vi "MovementModel.vi"(0 "Start Vector":T3, 2 "Destination":cluster{"x":dbl, "y":dbl}, 3 "Log All Points":bool, 5 "Segment Length (m)":dbl=0.1, 8 "Do Force Direction":bool, 9 "Movement Settings":T2={"Arrival Tolerance (m)"=0.01, "Closeness Threshold (m)"=0.5, "Pit Obstacle Radius (m)"=0.5, "Pit Locations"=[]}, 10 "Turn Radius (m)":dbl=1.7, 11 "Force Direction Forward (If Forcing)":bool) -> (15 "Move":T1, 18 "Final Position":cluster{"x":dbl, "y":dbl, "angle":dbl})   [LabVIEW 2015, in "Navigation2017.lvlib"]
doc: "Closeness Threshold is used to calculate closeness of each robot corner to walls and obstacles, which is summed and returned as Closeness Sum (a value used in path scoring).\n\nFrom lua prototype:\n--[[\nIteratively moves the robot along a circular/straight curve towards the \nend point. This movement may or may not succeed, and the result is given\nin didReach. The \"resolution\" of the movement is determined by segLength,\nin meters/iteration of movement. The movement will also fail if the robot \ncollides with the edge of the arena. \n\nThe robot may move forward or backward, depending on the closer of the \nsummed distances of the cameras on the front and back.\n\nTurning radius is determined by the variable provided above.\n\nlogAllPoints defaults to false\n \nParams:\n startX, startY - in meters\n startAngle - in rads\n destX, destY - destination point\n (you cannot specify an end angle, fundamentally)\n logAllPoints - for animation and rendering. defaults to false if set to nil\n forceDirection - force robot to move forwards or backwards. nil lets closer end \n of robot determine. Forwards = true, backwards = false if you do set this\n value.\n\nReturns a movement table:\n- didReach\n- didCollide\n- angleSum (how many radians robot turned over course of movement)\n- length (sum length of segments)\n- closeness (closeness of robot to walls and pits. should be mostly independent of segLength)\n- array of positions: (either just a couple or many, depending on logAllPoints)\n - {x, y, angle}\n- movedFwd (boolean)\n--]]"
uses:
  Navigation2017.lvlib
  Vector.ctl
  MovementSettings.ctl
  Move.ctl
  <vilib>/Analysis/coordinate.llb/Angle Range (Degree).ctl
  <vilib>/Analysis/coordinate.llb/Wrap Angle (scalar).vi
  Navigation2017-SubVIs.lvlib
  Navigation2017-util.lvlib
  <vilib>/Analysis/NI_AAL_Angle.lvlib
panel:
  # "OUTPUTS"
  # "INPUTS"
  # "Analogous to \nmovementmodel.lua -> move()"
  # "--[[\nIteratively moves the robot along a circular/straight curve towards the \nend point. This movement may or may not succeed, and the result is given\nin didReach. The \"resolution\" of the movement is determined by segLength,\nin meters/iteration of movement. The movement will also fail if the robot \ncollides with the edge of the arena. \n\nThe robot may move forward or backward, depending on the closer of the \nsummed distances of the cameras on the front and back.\n\nTurning radius is determined by the variable provided above.\n\nlogAllPoints defaults to false\n    \nParams:\n  startX, startY - in meters\n  startAngle - in rads\n  destX, destY - destination point\n    (you cannot specify an end angle, fundamentally)\n  logAllPoints - for animation and rendering. defaults to false if set to nil\n  forceDirection - force robot to move forwards or backwards. nil lets closer end \n    of robot determine. Forwards = true, backwards = false if you do set this\n    value.\n\nReturns a movement table:\n- didReach\n- didCollide\n- angleSum (how many radians robot turned over course of movement)\n- length (sum length of segments)\n- closeness (closeness of robot to walls and pits. should be mostly independent of segLength)\n- array of positions: (either just a couple or many, depending on logAllPoints)\n  - {x, y, angle}\n- movedFwd (boolean)\n--]]"
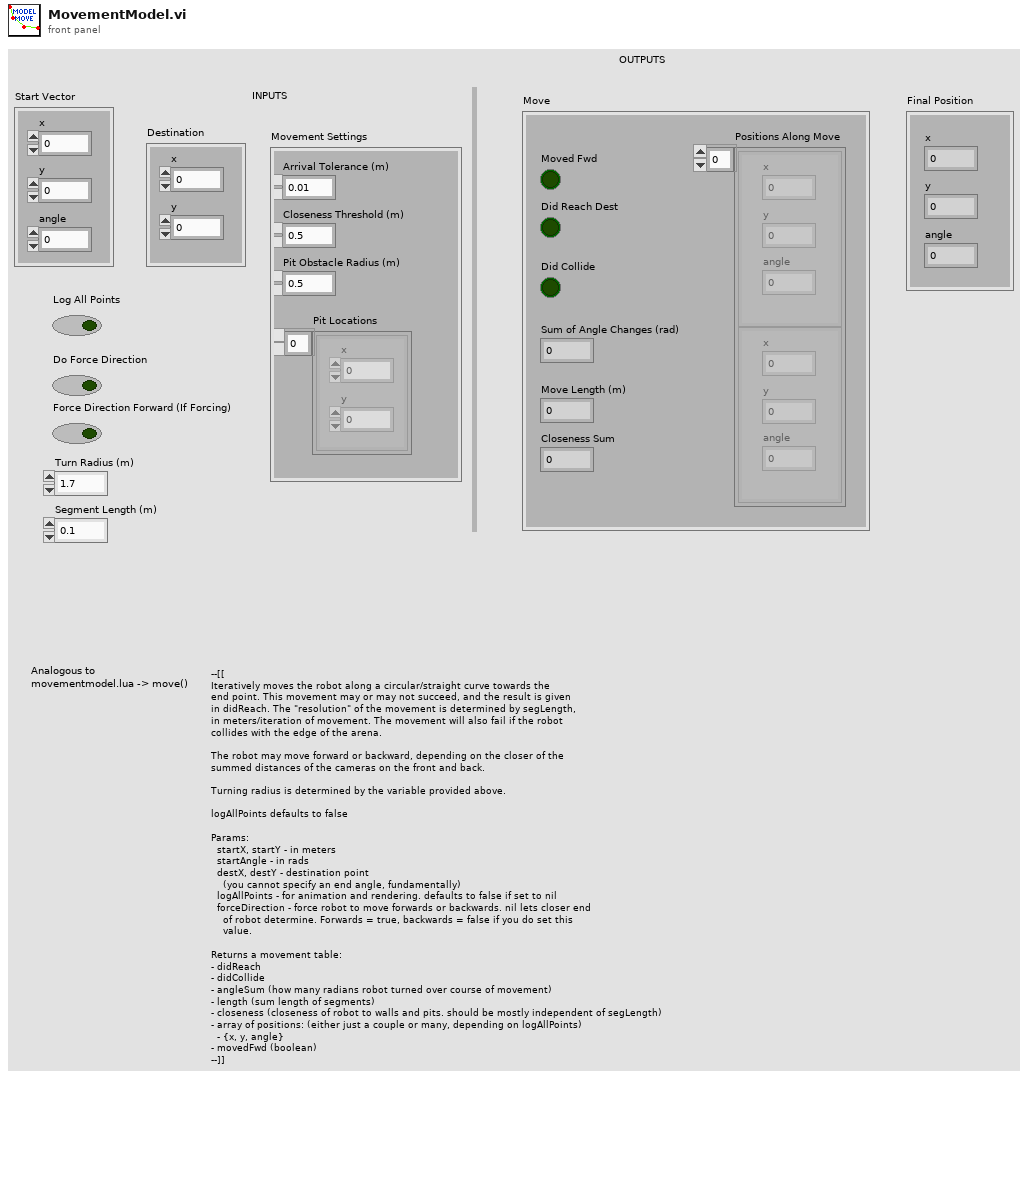
[diagram p1: front panel]
types:
  T1 = typedef "Navigation2017.lvlib/Move.ctl" = cluster{"Did Reach Dest":bool, "Did Collide":bool, "Sum of Angle Changes (rad)":dbl, "Move Length (m)":dbl, "Closeness Sum":dbl, "Positions Along Move":cluster{"x":dbl, "y":dbl, "angle":dbl}[], "Moved Fwd":bool}
  T2 = typedef "Navigation2017.lvlib/MovementSettings.ctl" = cluster{"Arrival Tolerance (m)":dbl, "Closeness Threshold (m)":dbl, "Pit Obstacle Radius (m)":dbl, "Pit Locations":cluster{"x":dbl, "y":dbl}[]}
  T3 = typedef "Navigation2017.lvlib/Vector.ctl" = cluster{"x":dbl, "y":dbl, "angle":dbl}
  T4 = typedef "NI_AAL_Angle.lvlib/Angle Range (Degree).ctl" = u16
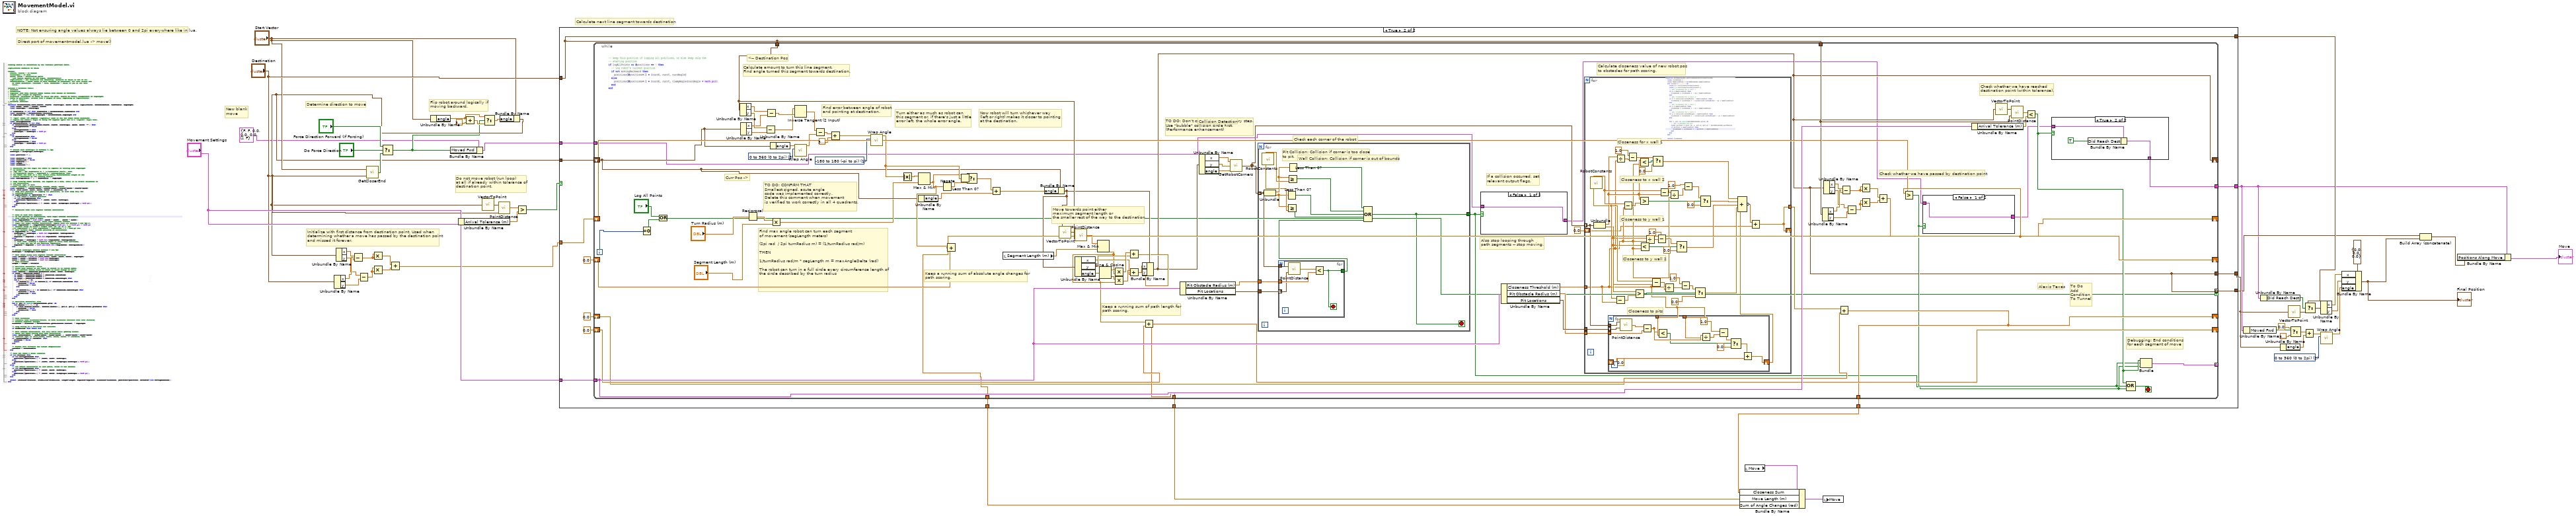
[diagram p0: block diagram]
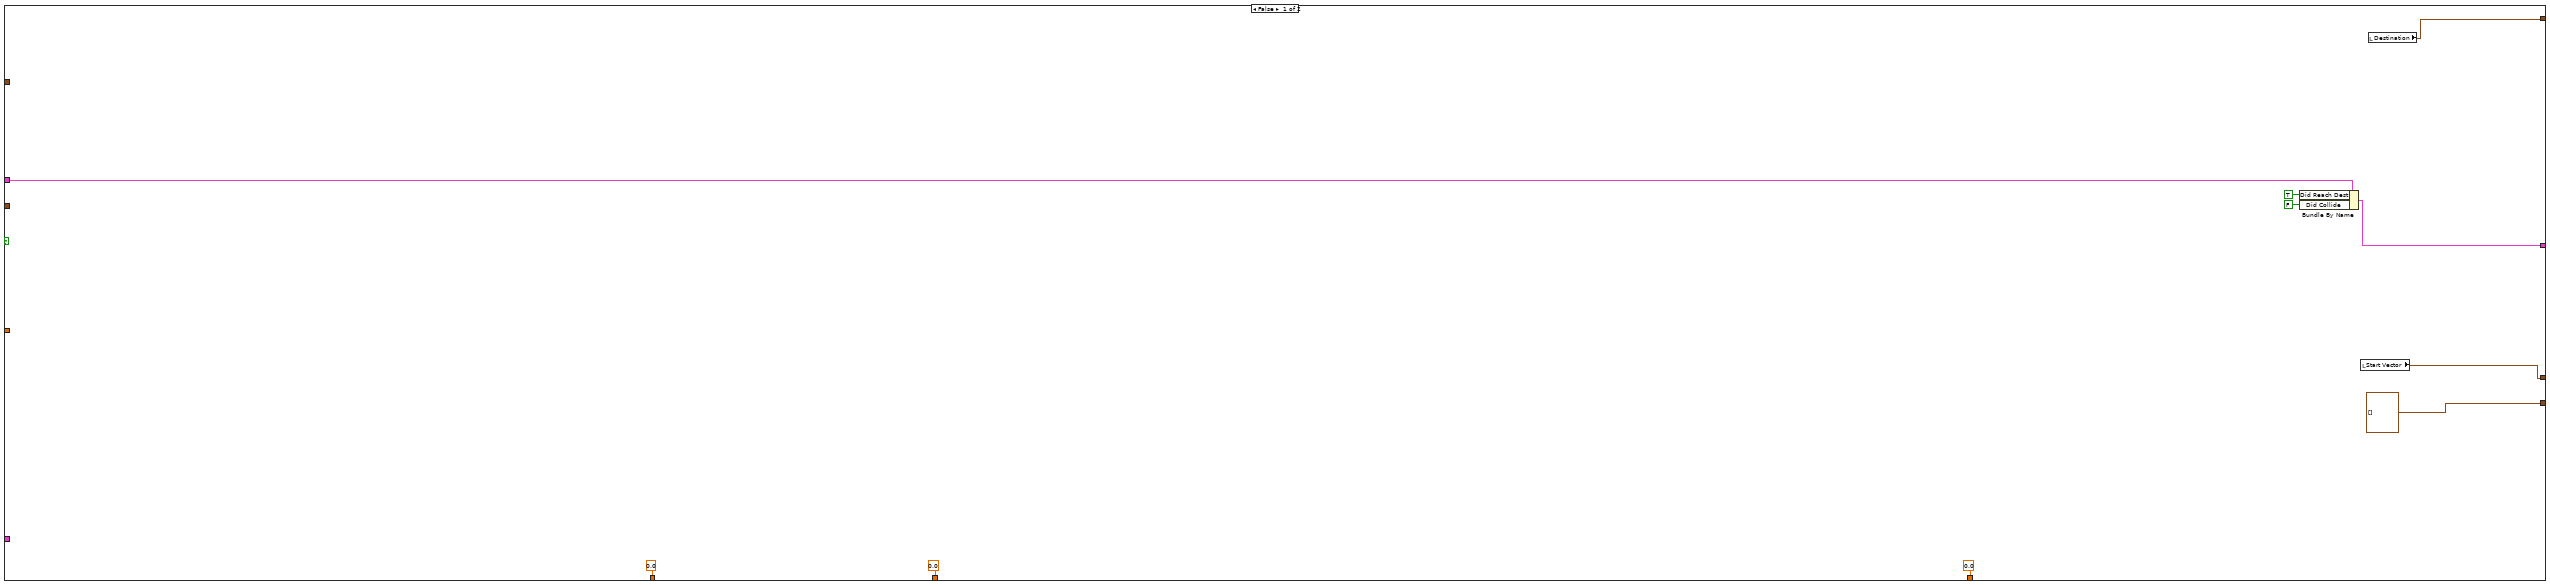
[diagram p2: hidden frame]
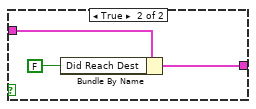
[diagram p4: hidden frame]
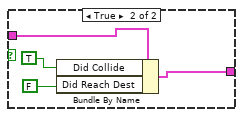
[diagram p5: hidden frame]
diagram:
  w36 = T4 2 items=["none", "-180 to 180 (-pi to pi)", "0 to 360 (0 to 2pi)"] ("angle range")
  # "New blank\nmove"
  # "Initialize with first distance from destination point. Used when\ndetermining whether a move has passed by the destination point\nand missed it forever."
  # "Do not move robot (run loop)\nat all if already within tolerance of \ndestination point."
  # "Calculate next line segment towards destination"
  # "NOTE: Not ensuring angle values always lie between 0 and 2pi everywhere like in lua."
  # "Flip robot around logically if\nmoving backward."
  # "Determine direction to move"
  # "Direct port of movementmodel.lua -> move()"
  n1 = Unbundle By Name("Destination") -> ("x"=w29:dbl, "y"=w25:dbl)
  n2 = call "GetCloserEnd.vi"("Destination"="Destination", "Robot Pos"="Start Vector") -> ("Forward Closer"=w51:bool)
  n3 = Select(t="Force Direction Forward (If Forcing)", s="Do Force Direction", f=w51) -> (s? t:f=w6:bool)
  n4 = Unbundle By Name("Start Vector") -> ("angle"=w17:dbl)
  n5 = Bundle By Name(cluster=T1 {"Did Reach Dest"=FALSE, "Did Collide"=FALSE, "Sum of Angle Changes (rad)"=0.0, "Move Length (m)"=0.0, "Closeness Sum"=0.0, "Positions Along Move"=[], "Moved Fwd"=FALSE} ("Move"), "Moved Fwd"=w6) -> (w2:T1)
  n6 = Unbundle By Name("Movement Settings") -> ("Arrival Tolerance (m)"=w47:dbl)
  n7 = Add(x=w17, y=3.141592653589793) -> (x+y=w19:dbl)
  n8 = Select(t=w17, s=w6, f=w19) -> (s? t:f=w18:dbl)
  n9 = Bundle By Name(cluster="Start Vector", "angle"=w18) -> (w15:T3)
  n10 = Unbundle By Name(w15) -> ("x"=w30:dbl, "y"=w26:dbl)
  n11 = Subtract(x=w30, y=w29) -> (x-y=w28:dbl)
  n12 = Subtract(x=w26, y=w25) -> (x-y=w27:dbl)
  n13 = Multiply(x=w28, y=w28) -> (x*y=w24:dbl)
  n14 = Multiply(x=w27, y=w27) -> (x*y=w23:dbl)
  n15 = Add(x=w24, y=w23) -> (x+y=w22:dbl)
  n16 = call "VectorToPoint.vi"("Vector"=w15) -> ("Point"=w46:cluster{"x":dbl, "y":dbl})
  n17 = call "PointDistance.vi"("Point 2"="Destination", "Point 1"=w46) -> ("Distance"=w48:dbl)
  n18 = Greater?(x=w48, y=w47) -> (0:w49:bool)
  n19 = case shown="True" w49 {
    tunnel: w15 -> [_ w77]
    tunnel: [cluster{"x":dbl, "y":dbl, "angle":dbl}[] [] w66] -> w20
    tunnel: "Destination" -> [_ w73]
    tunnel: [0.0 w76] -> w7
    tunnel: [0.0 w75] -> w8
    tunnel: "Movement Settings" -> [_ w74]
    tunnel: [w59 w73] -> w44
    tunnel: [w58 w72] -> w39
    tunnel: [0.0 w71] -> w11
    tunnel: w22 -> [_ w67]
    tunnel: [w55 w65] -> w1
    tunnel: w2 -> [w54 w64]
    frame False {
      n20 = Bundle By Name(cluster=w54, "Did Reach Dest"=TRUE, "Did Collide"=FALSE) -> (w55:T1)
      n21 = local read "Start Vector"() -> (w58:T3)
      n22 = local read "Destination"() -> (w59:cluster{"x":dbl, "y":dbl})
    }
    frame True {
      n23 = while {
        tunnel: w73 -> [w164]
        tunnel: [w155] -> w76
        tunnel: [w159] -> w75
        tunnel: w74 -> [w163]
        tunnel: w73 -> [w162]
        tunnel: [w86] -> w72
        tunnel: [w157] -> w71
        shift-right: [w159] -> _
        shift-left: 0.0 -> [w160]
        shift-right: [w157] -> _
        shift-left: 0.0 -> [w158]
        shift-right: [w155] -> _
        shift-left: 0.0 -> [w156]
        shift-right: [w154] -> _
        shift-left: w67 -> [w153]
        tunnel: [w88] -> _ mode=indexing
        tunnel: [w86] -> w66 mode=indexing if=w82
        shift-right: [w86] -> _
        shift-left: w77 -> [w85]
        tunnel: [w80] -> w65
        tunnel: w64 -> [w79]
        i -> [w165]
        stop <- w161 stop-if-true
        w104 = T4 1 items=["none", "-180 to 180 (-pi to pi)", "0 to 360 (0 to 2pi)"] ("angle range")
        w151 = T4 2 items=["none", "-180 to 180 (-pi to pi)", "0 to 360 (0 to 2pi)"] ("angle range")
        # "Debugging: End conditions\nfor each segment of move"
        # "To Do\nAdd\nCondition\nTo Tunnel"
        # "Alexis Texas"
        # "Check whether we have reached\ndestination point (within tolerance)."
        # "Check whether we have passed by destination point"
        # "Calculate closeness value of new robot pos\nto obstacles for path scoring."
        # "Also stop looping through\npath segments -- stop moving."
        # "If a collision occurred, set\nrelevant output flags."
        # "Check each corner of the robot"
        # "TO DO: Don't calculate corners every step. \nUse \"bubble\" collision circle first.\n(Performance enhancement)"
        # "Collision Detection"
        # "Keep a running sum of path length for\npath scoring."
        # "Move towards point either\nmaximum segment length or\nthe smaller rest of the way to the destination."
        # "Keep a running sum of absolute angle changes for\npath scoring."
        # "<-- Destination Pos"
        # "Now robot will turn whichever way\n(left or right) makes it closer to pointing\nat the destination."
        # "TO DO: CONFIRM THAT\nSmallest signed, acute angle\ncode was implemented correctly.\nDelete this comment when movement\nis verified to work correctly in all 4 quadrants."
        # "Turn either as much as robot can\nthis segment or, if there's just a little \nerror left, the whole error angle."
        # "Find error between angle of robot\nand pointing at destination."
        # "Curr Pos ->"
        # "Calculate amount to turn this line segment.\nFind angle turned this segment towards destination."
        # "Find max angle robot can turn each segment\nof movement (segLength meters)\n\n(2pi rad  / 2pi turnRadius m) = (1/turnRadius rad/m)\n\nTHEN\n\n1/turnRadius rad/m * segLength m = maxAngleDelta (rad)\n\nThe robot can turn in a full circle every circumference length of\nthe circle described by the turn radius"
        n24 = Equal To 0?(x=w165) -> (x = 0?=w92:bool)
        n25 = Or(x="Log All Points", y=w92) -> (x .or. y?=w82:bool)
        n26 = Unbundle By Name(w164) -> ("x"=w150:dbl, "y"=w149:dbl)
        n27 = Unbundle By Name(w85) -> ("x"=w148:dbl, "y"=w147:dbl)
        n28 = Reciprocal(x="Turn Radius (m)") -> (1/x=w142:dbl)
        n29 = Subtract(x=w149, y=w147) -> (x-y=w145:dbl)
        n30 = Subtract(x=w150, y=w148) -> (x-y=w146:dbl)
        n31 = Unbundle By Name(w85) -> ("angle"=w152:dbl)
        n32 = Multiply(x=w142, y="Segment Length (m)") -> (x*y=w84:dbl)
        n33 = Inverse Tangent (2 Input)(1:w146, 2:w145) -> (0:w109:dbl)
        n34 = call-poly <vilib>:"Wrap Angle.vi"("angle range"=w151, "angle in"=w152) -> ("angle out"=w108:dbl)  [unwired: 8 in, 1 out]
        n35 = Subtract(x=w109, y=w108) -> (x-y=w107:dbl)
        n36 = Add(x=w107, y=3.141592653589793) -> (x+y=w105:dbl)
        n37 = call-poly <vilib>:"Wrap Angle.vi"("angle range"=w104, "angle in"=w105) -> ("angle out"=w100:dbl)  [unwired: 8 in, 1 out]
        n38 = Absolute Value(x=w100) -> (abs(x)=w103:dbl)
        n39 = Max & Min(x=w103, y=w84) -> (min(x,y)=w96:dbl)  [unwired: 1 out]
        n40 = Unbundle By Name(w85) -> ("angle"=w102:dbl)
        n41 = Negate(x=w96) -> (-x=w99:dbl)
        n42 = Add(x=w96, y=w156) -> (x+y=w155:dbl)
        n43 = Less Than 0?(x=w100) -> (x < 0?=w101:bool)
        n44 = Select(t=w96, s=w101, f=w99) -> (s? t:f=w98:dbl)
        n45 = Add(x=w98, y=w102) -> (x+y=w97:dbl)
        n46 = local read "Segment Length (m)"() -> (w83:dbl)
        n47 = Bundle By Name(cluster=w85, "angle"=w97) -> (w132:T3)
        n48 = call "VectorToPoint.vi"("Vector"=w132) -> ("Point"=w141:cluster{"x":dbl, "y":dbl})
        n49 = call "PointDistance.vi"("Point 2"=w164, "Point 1"=w141) -> ("Distance"=w140:dbl)
        n50 = Unbundle By Name(w132) -> ("x"=w133:dbl, "y"=w134:dbl, "angle"=w135:dbl)
        n51 = Max & Min(x=w140, y=w83) -> (min(x,y)=w131:dbl)  [unwired: 1 out]
        n52 = Sine & Cosine(0:w135) -> (1:w139:dbl, 2:w138:dbl)
        n53 = Multiply(x=w139, y=w131) -> (x*y=w137:dbl)
        n54 = Multiply(x=w138, y=w131) -> (x*y=w136:dbl)
        n55 = Add(x=w137, y=w134) -> (x+y=w129:dbl)
        n56 = Add(x=w136, y=w133) -> (x+y=w130:dbl)
        n57 = Bundle By Name(cluster=w132, "x"=w130, "y"=w129) -> (w86:T3)
        n58 = Add(x=w131, y=w160) -> (x+y=w159:dbl)
        n59 = Unbundle By Name(w163) -> ("Pit Obstacle Radius (m)"=w125:dbl, "Pit Locations"=w124:cluster{"x":dbl, "y":dbl}[])
        n60 = Unbundle By Name(w86) -> ("x"=w128:dbl, "y"=w127:dbl, "angle"=w126:dbl)
        n61 = call "GetRobotCorners.vi"("botAngle (rad)"=w126, "botY (m)"=w127, "botX (m)"=w128) -> ("Corner Points (m)"=w123:cluster{dbl, dbl}[])
        n62 = for {
          tunnel: w123 -> [w239] mode=indexing
          tunnel: w125 -> [w238]
          tunnel: w124 -> [w237]
          tunnel: [w235] -> w89
          stop <- w235 stop-if-true
          # "Pit Collision: Collision if corner is too close\nto pit."
          # "Wall Collision: Collision if corner is out of bounds"
          n63 = call "RobotConstants.vi"() -> ("Arena Width (m)"=w247:dbl, "Arena Height (m)"=w245:dbl)  [unwired: 3 out]
          n64 = Unbundle(w239) -> (w246:dbl, w244:dbl)
          n65 = for {
            tunnel: w239 -> [w252]
            tunnel: w238 -> [w250]
            tunnel: w237 -> [w249] mode=indexing
            tunnel: [w248] -> w236
            stop <- w248 stop-if-true
            n66 = call "PointDistance.vi"("Point 2"=w249, "Point 1"=w252) -> ("Distance"=w251:dbl)
            n67 = Less?(x=w251, y=w250) -> (x < y?=w248:bool)
          }
          n68 = Less Than 0?(x=w244) -> (x < 0?=w241:bool)
          n69 = Greater Or Equal?(x=w244, y=w245) -> (x >= y?=w240:bool)
          n70 = Greater Or Equal?(x=w246, y=w247) -> (x >= y?=w242:bool)
          n71 = Less Than 0?(x=w246) -> (x < 0?=w243:bool)
          n72 = Compound Arithmetic op=OR(w243, w242, w241, w240, w236) -> (w235:bool)
        }
        n73 = case shown="False" w89 {
          tunnel: w79 -> [w230 w232]
          tunnel: [w230 w231] -> w78
          frame False {
          }
          frame True {
            n74 = Bundle By Name(cluster=w232, "Did Collide"=TRUE, "Did Reach Dest"=FALSE) -> (w231:T1)
          }
        }
        n75 = Unbundle By Name(w163) -> ("Closeness Threshold (m)"=w122:dbl, "Pit Obstacle Radius (m)"=w120:dbl, "Pit Locations"=w121:cluster{"x":dbl, "y":dbl}[])
        n76 = for {
          tunnel: w123 -> [w181] mode=indexing
          tunnel: w122 -> [w178]
          tunnel: [w176] -> w111
          tunnel: w121 -> [w180]
          tunnel: w120 -> [w179]
          shift-right: [w176] -> _
          shift-left: 0.0 -> [w177]
          # "Closeness to pits"
          # "Closeness to y wall 2"
          # "Closeness to y wall 1"
          # "Closeness to x wall 2"
          # "Closeness for x wall 1"
          n77 = call "RobotConstants.vi"() -> ("Arena Width (m)"=w202:dbl, "Arena Height (m)"=w183:dbl)  [unwired: 3 out]
          n78 = Unbundle(w181) -> (w201:dbl, w182:dbl)
          n79 = for {
            tunnel: w181 -> [w229]
            tunnel: w180 -> [w228] mode=indexing
            tunnel: w179 -> [w226]
            tunnel: w178 -> [w225]
            tunnel: w178 -> [w221]
            shift-right: [w215] -> w174
            shift-left: 0.0 -> [w216]
            n80 = call "PointDistance.vi"("Point 2"=w228, "Point 1"=w229) -> ("Distance"=w227:dbl)
            n81 = Subtract(x=w227, y=w226) -> (x-y=w222:dbl)
            n82 = Less?(x=w222, y=w225) -> (x < y?=w220:bool)
            n83 = Divide(x=w222, y=w221) -> (x/y=w223:dbl)
            n84 = Subtract(x=1.0, y=w223) -> (x-y=w219:dbl)
            n85 = Select(t=w219, s=w220, f=0.0) -> (s? t:f=w217:dbl)
            n86 = Add(x=w217, y=w216) -> (x+y=w215:dbl)
          }
          n87 = Subtract(x=w183, y=w178) -> (x-y=w185:dbl)
          n88 = Divide(x=w201, y=w178) -> (x/y=w210:dbl)
          n89 = Subtract(x=w202, y=w178) -> (x-y=w209:dbl)
          n90 = Subtract(x=1.0, y=w210) -> (x-y=w211:dbl)
          n91 = Greater?(x=w182, y=w185) -> (0:w191:bool)
          n92 = Less?(x=w201, y=w178) -> (x < y?=w214:bool)
          n93 = Greater?(x=w201, y=w209) -> (0:w208:bool)
          n94 = Less?(x=w182, y=w178) -> (x < y?=w197:bool)
          n95 = Divide(x=w182, y=w178) -> (x/y=w194:dbl)
          n96 = Subtract(x=w183, y=w182) -> (x-y=w184:dbl)
          n97 = Select(t=w211, s=w214, f=0.0) -> (s? t:f=w200:dbl)
          n98 = Subtract(x=1.0, y=w194) -> (x-y=w195:dbl)
          n99 = Subtract(x=w202, y=w201) -> (x-y=w203:dbl)
          n100 = Divide(x=w184, y=w178) -> (x/y=w187:dbl)
          n101 = Divide(x=w203, y=w178) -> (x/y=w204:dbl)
          n102 = Select(t=w195, s=w197, f=0.0) -> (s? t:f=w192:dbl)
          n103 = Subtract(x=1.0, y=w187) -> (x-y=w189:dbl)
          n104 = Subtract(x=1.0, y=w204) -> (x-y=w206:dbl)
          n105 = Select(t=w189, s=w191, f=0.0) -> (s? t:f=w186:dbl)
          n106 = Select(t=w206, s=w208, f=0.0) -> (s? t:f=w199:dbl)
          n107 = Compound Arithmetic op=ADD(w200, w199, w192, w186, w174) -> (invert w198:dbl)
          n108 = Add(x=w198, y=w177) -> (x+y=w176:dbl)
        }
        n109 = Unbundle By Name(w162) -> ("x"=w118:dbl, "y"=w114:dbl)
        n110 = Unbundle By Name(w86) -> ("x"=w119:dbl, "y"=w115:dbl)
        n111 = Add(x=w111, y=w158) -> (x+y=w157:dbl)
        n112 = Subtract(x=w119, y=w118) -> (x-y=w117:dbl)
        n113 = Subtract(x=w115, y=w114) -> (x-y=w116:dbl)
        n114 = Multiply(x=w117, y=w117) -> (x*y=w113:dbl)
        n115 = Multiply(x=w116, y=w116) -> (x*y=w112:dbl)
        n116 = Add(x=w113, y=w112) -> (x+y=w154:dbl)
        n117 = Greater?(x=w154, y=w153) -> (0:w90:bool)
        n118 = case shown="False" w90 {
          tunnel: w78 -> [w170 w172]
          tunnel: [w170 w171] -> w81
          frame False {
          }
          frame True {
            n119 = Bundle By Name(cluster=w172, "Did Reach Dest"=FALSE) -> (w171:T1)
          }
        }
        n120 = Unbundle By Name(w163) -> ("Arrival Tolerance (m)"=w94:dbl)
        n121 = call "VectorToPoint.vi"("Vector"=w86) -> ("Point"=w93:cluster{"x":dbl, "y":dbl})
        n122 = call "PointDistance.vi"("Point 2"=w162, "Point 1"=w93) -> ("Distance"=w95:dbl)
        n123 = Less?(x=w95, y=w94) -> (x < y?=w91:bool)
        n124 = case shown="True" w91 {
          tunnel: w81 -> [w166 w168]
          tunnel: [w166 w167] -> w80
          frame False {
          }
          frame True {
            n125 = Bundle By Name(cluster=w168, "Did Reach Dest"=TRUE) -> (w167:T1)
          }
        }
        n126 = Compound Arithmetic op=OR(w91, w90, w89) -> (w161:bool)
        n127 = Bundle(w91, w90, w89) -> (w88:cluster{bool, bool, bool})  [unwired: 1 in]
      }
    }
  }
  n128 = local read "Move"() -> (w9:T1)
  n129 = Bundle By Name(cluster=w9, "Closeness Sum"=w11, "Move Length (m)"=w8, "Sum of Angle Changes (rad)"=w7) -> (w10:T1)
  n130 = local write "Move"(w10) -> ()
  n131 = Unbundle By Name(w1) -> ("Moved Fwd"=w13:bool)
  n132 = Unbundle By Name(w1) -> ("Did Reach Dest"=w12:bool)
  n133 = Unbundle By Name(w39) -> ("angle"=w38:dbl)
  n134 = call "VectorToPoint.vi"("Vector"=w39) -> ("Point"=w43:cluster{"x":dbl, "y":dbl})
  n135 = Select(t=0.0, s=w13, f=3.141592653589793) -> (s? t:f=w40:dbl)
  n136 = Add(x=w40, y=w38) -> (x+y=w37:dbl)
  n137 = Select(t=w44, s=w12, f=w43) -> (s? t:f=w34:cluster{"x":dbl, "y":dbl})
  n138 = call-poly <vilib>:"Wrap Angle.vi"("angle range"=w36, "angle in"=w37) -> ("angle out"=w35:dbl)  [unwired: 8 in, 1 out]
  n139 = Unbundle By Name(w34) -> ("x"=w33:dbl, "y"=w32:dbl)
  n140 = Bundle By Name(cluster=T3 {"x"=0.0, "y"=0.0, "angle"=0.0} ("Vector"), "x"=w33, "y"=w32, "angle"=w35) -> (w31:T3)
  "Final Position" <- w31
  n141 = Build Array (concatenate)(w20, w31) -> (w14:T3[])
  n142 = Bundle By Name(cluster=w1, "Positions Along Move"=w14) -> (→"Move":T1)
